vi "Get Flattened Message.vi"(8 "error in (no error)":errorcluster, 11 "Message in":refnum<class "Message.lvclass">) -> (0 "error out":errorcluster, 2 "Flattened Message":string, 3 "Message out":refnum<class "Message.lvclass">)   [LabVIEW 2020, in "Stream-Simple-Msg.lvlib" / "Message.lvclass"]
uses:
  Message.lvclass
  Message Data.ctl
  Message.lvclass/Message.ctl
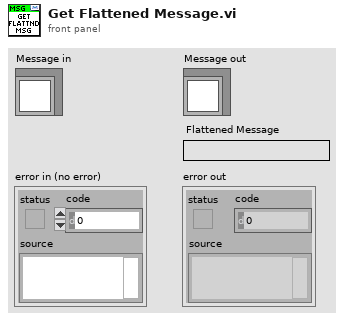
[diagram p1: front panel]
types:
  T1 = typedef "Stream-Simple-Msg.lvlib/Message.lvclass/Message Data.ctl" = cluster{"ID":string, "Data":string}
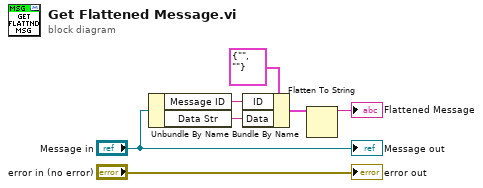
[diagram p0: block diagram]
diagram:
  n1 = Unbundle By Name("Message in") -> ("Message ID"=w4:string, "Data Str"=w3:string)
  n2 = Bundle By Name(cluster=T1 {"ID"="", "Data"=""} ("Message Data"), "ID"=w4, "Data"=w3) -> (w2:T1)
  n3 = Flatten To String(anything=w2) -> (data string=→"Flattened Message":string)  [unwired: 3 in, 2 out]
  "error out" <- "error in (no error)"
  "Message out" <- "Message in"
